vi "CumSum.vi"(1 "Array":dbl[](array[numeric])) -> (0 "CumSum":dbl[](array[numeric]))   [LabVIEW 2020]
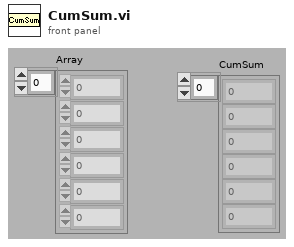
[diagram p1: front panel]
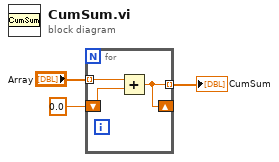
[diagram p0: block diagram]
diagram:
  n1 = for {
    tunnel: "Array" -> [w5] mode=indexing
    tunnel: [w4] -> w1 mode=indexing
    shift-right: [w4] -> _
    shift-left: 0.0 -> [w6]
    n2 = Add(x=w5, y=w6) -> (x+y=w4:dbl)
  }
  "CumSum" <- w1
